vi "random number & chart.vi"() -> ()   [LabVIEW 2017]
panel:
  out "number (0 to 1)":dbl
  out "Numeric":i32
  in  "stop":bool
  out "Waveform Graph":dbl[](graph)
  out "Waveform Chart":dbl(graph)
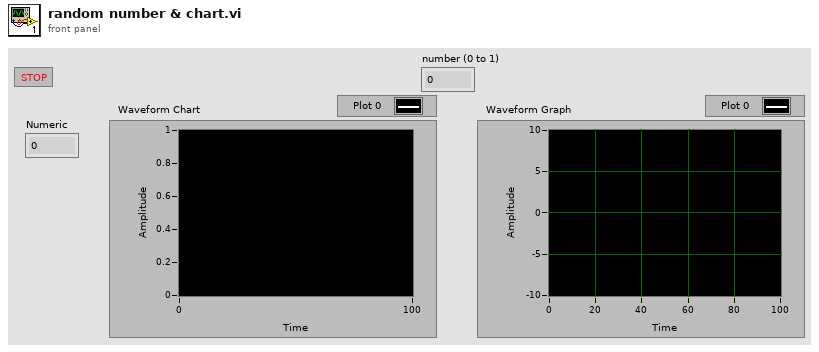
[diagram p1: front panel]
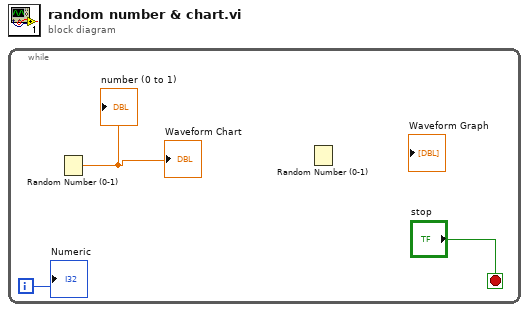
[diagram p0: block diagram]
diagram:
  n1 = while {
    i -> [w1]
    stop <- "stop" stop-if-true
    n2 = Random Number (0-1)() -> (number: 0 to 1=→"Waveform Chart" →"number (0 to 1)":dbl)
    n3 = Random Number (0-1)() -> ()  [unwired: 1 out]
    "Numeric" <- w1
  }
